vi "daemon.vi"(7 "Watchdog":refnum<notifier>, 10 "args":variant, 11 "Buffer":refnum<queue>) -> ()   [LabVIEW 2024, in "ConsoleWriter.lvclass"]
uses:
  ConsoleWriter.lvclass
panel:
  out "Console":string
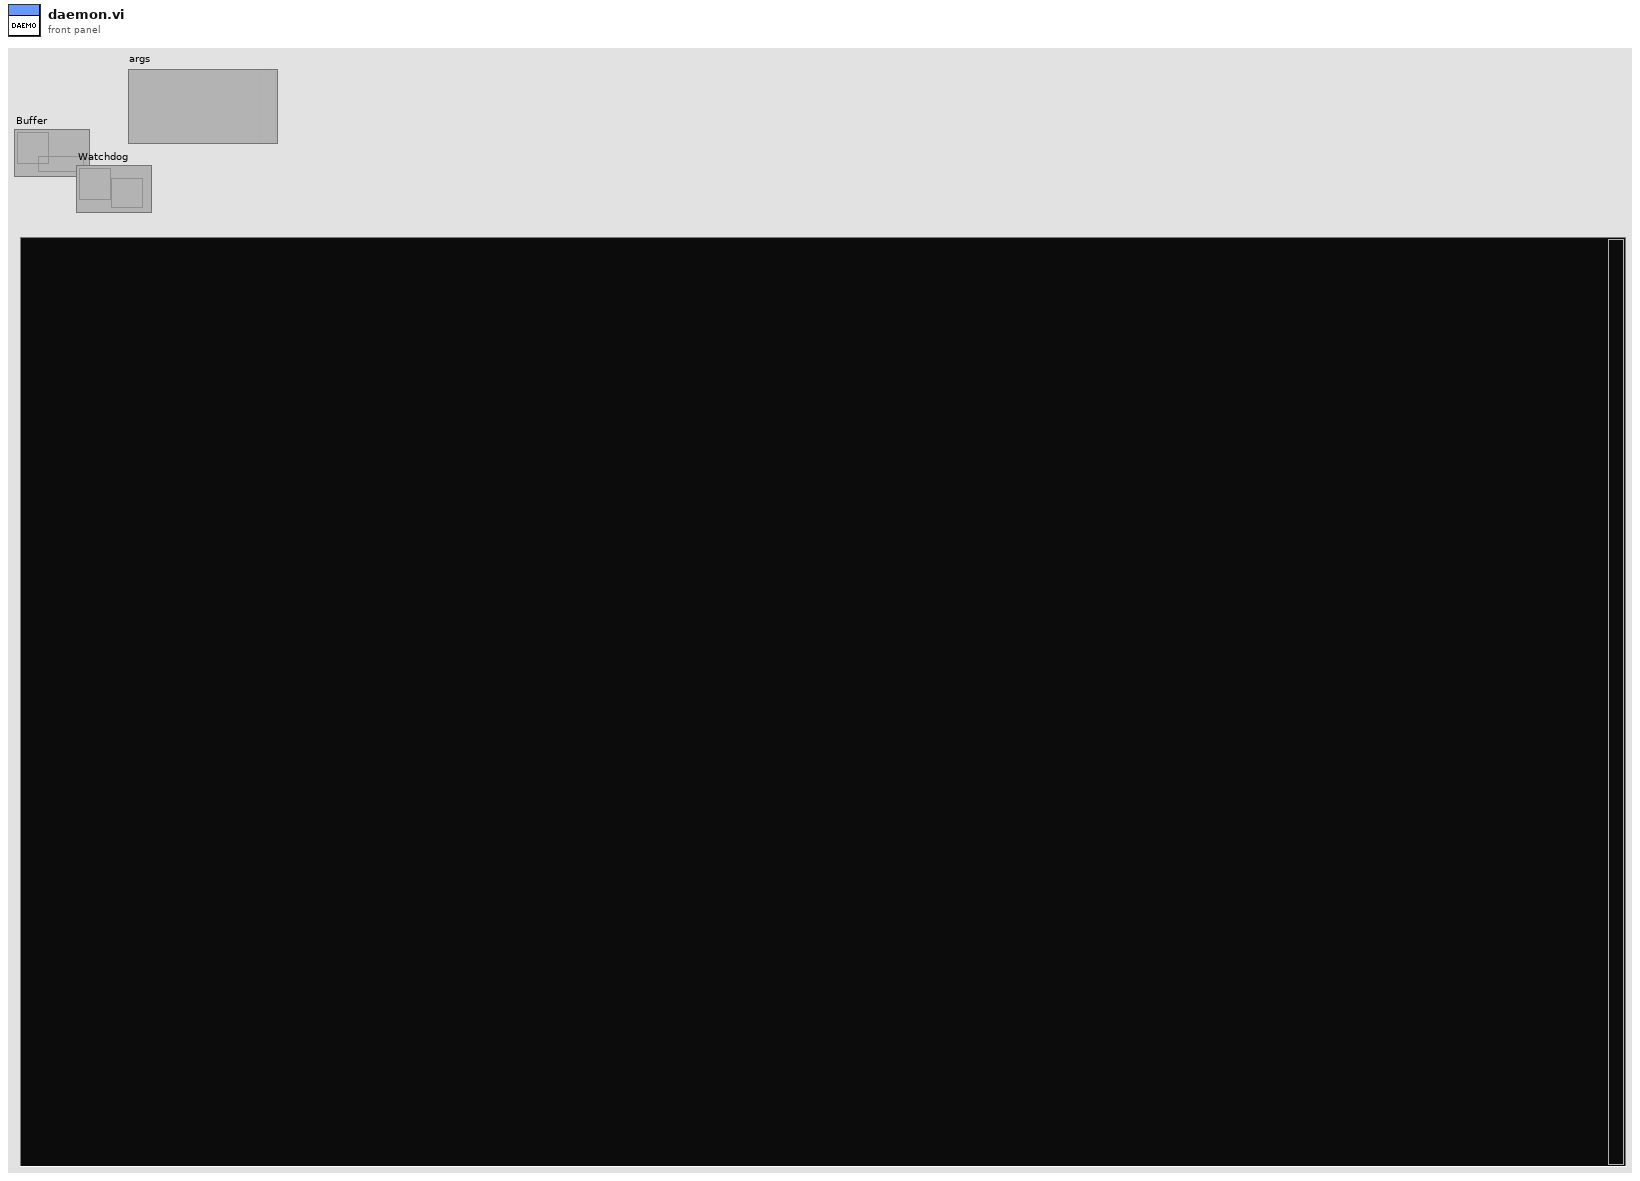
[diagram p1: front panel]
types:
  T1 = enum32{"Invalid", "Standard", "Closed", "Hidden", "Minimized", "Maximized"}
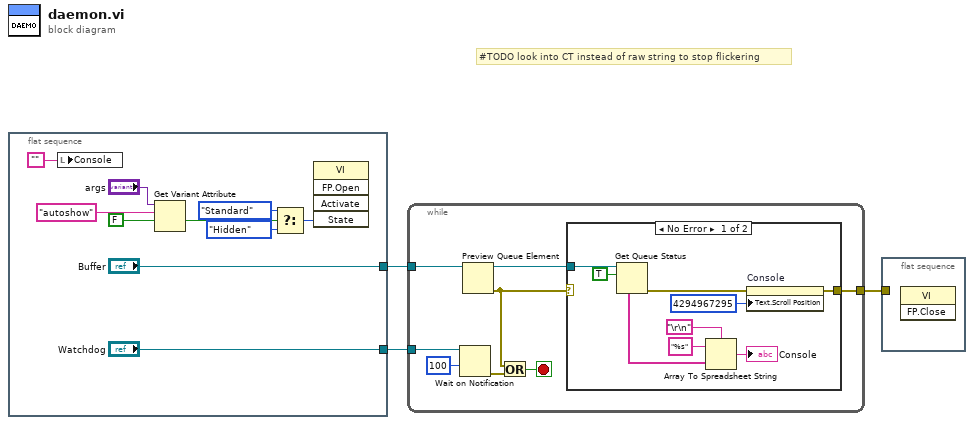
[diagram p0: block diagram]
diagram:
  # "#TODO look into CT instead of raw string to stop flickering"
  n1 = flat-sequence {
    tunnel: ["Buffer"] -> w3
    tunnel: ["Watchdog"] -> w1
    frame #0 {
      n2 = local write "Console"("") -> ()
      n3 = Get Variant Attribute(Variant="args", name="autoshow", default value (empty Variant)=FALSE) -> (value=w8:bool)  [unwired: 1 in, 3 out]
      n4 = Select(t=T1."Standard" ("State"), s=w8, f=T1."Hidden" ("State")) -> (s? t:f=w5:T1)
      n5 = invoke class="VI" method="FP.Open"("State"=w5) -> ()  [unwired: 4 in, 5 out]
    }
  }
  n6 = while {
    tunnel: w3 -> [w19]
    tunnel: [w21] -> w2
    tunnel: w1 -> [w18]
    stop <- w16 stop-if-true
    n7 = Wait on Notification(notifier=w18, timeout in ms (-1)=100) -> (error out=w15:errorcluster)  [unwired: 2 in, 3 out]
    n8 = Preview Queue Element(queue=w19) -> (queue out=w20:refnum<queue>, error out=w14:errorcluster)  [unwired: 2 in, 2 out]
    n9 = Or(x=w14, y=w15) -> (x .or. y?=w16:bool)
    n10 = case shown="No Error" w14 {
      selector: w14 -> [_ w30]
      tunnel: w20 -> [w29 _]
      tunnel: [w27 w30] -> w21
      frame No Error {
        n11 = Get Queue Status(queue=w29, return elements? (F)=TRUE) -> (error out=w27:errorcluster, elements=w22:string[])  [unwired: 1 in, 6 out]
        n12 = Array To Spreadsheet String(delimiter (Tab)="\r\n", array=w22, 3:"%s" ("format string")) -> (spreadsheet string=→"Console":string)
        n13 = property on="Console" class="Str"(error in=w27, "Text.Scroll Position"=u32 4294967295) -> ()  [unwired: 1 in, 2 out]
      }
      frame Error {
      }
    }
  }
  n14 = flat-sequence {
    tunnel: w2 -> [_]
    frame #0 {
      n15 = invoke class="VI" method="FP.Close"() -> ()  [unwired: 3 in, 3 out]
    }
  }
